vi "LINX - BlinkM Smart LED.vi"() -> ()   [LabVIEW 2020]
doc: "Set the color of a BlinkM Smart LED."
uses:
  vi.lib/MakerHub/LINX/LMH-LINX.lvlib
  vi.lib/MakerHub/LINX/Private/Device/Device.lvlib
  vi.lib/MakerHub/LINX/Public/Sensors/Lights/BlinkM/BlinkM.lvlib
  vi.lib/MakerHub/LINX/Public/Utilities/Open Serial.vi
panel:
  in  "I2C Channel":u8
  out "Loop Rate (Hz)":u32
  in  "Serial Port":refnum<visa-resource-name>
  in  "Stop Button":bool
  out "LED Color":u32(colorbox)
  in  "Blue":u8(slide) scale=0.0..255.0
  in  "Green":u8(slide) scale=0.0..255.0
  in  "Red":u8(slide) scale=0.0..255.0
  # "Circuit Schematic"
  # "LINX Device Settings"
  # "BlinkM Color"
  # "BlinkM Smart LED Example\n\nThis example demonstrates how to set the color of a BlinkM smart LED and assumes\nthe BlinkM is connected to I2C channel 0 and is the only device on the bus.\n\nNote: This example is configured to use a serial interface but can easily be modified\nto use TCP or run on myRIO.\n\nInstructions\n1. Select the COM Port associated with the LINX Device.\n2. Click the Run Arrow.\n3. Adjust the Red Green and Blue sliders to change the BlinkM color."
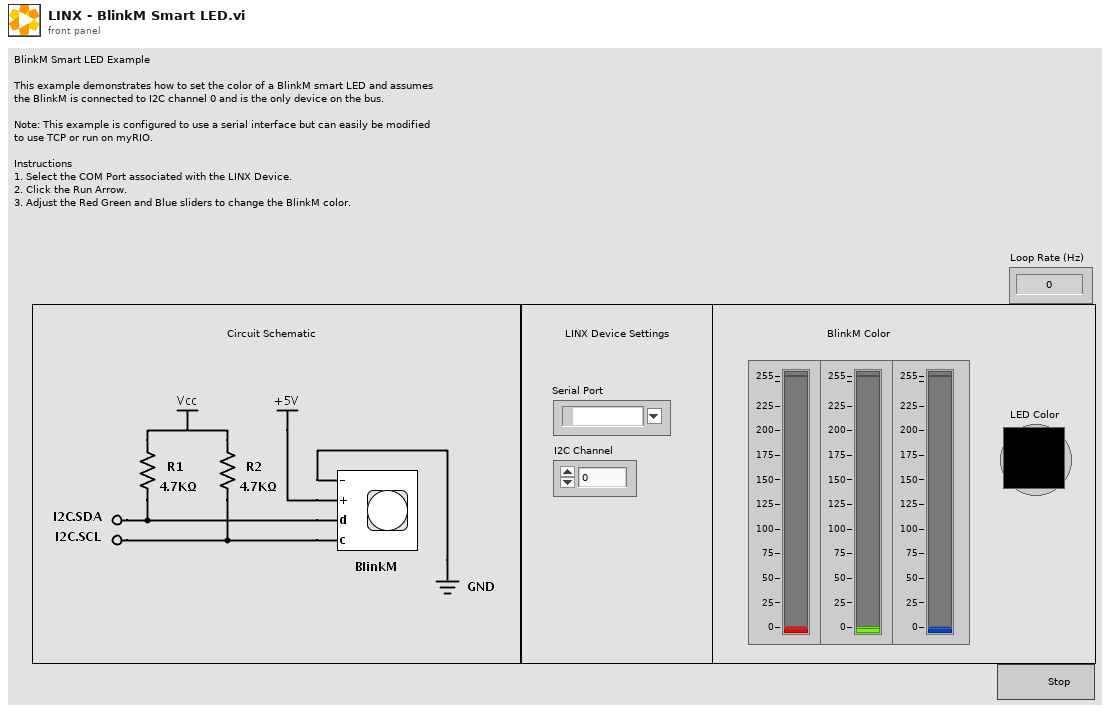
[diagram p1: front panel]
types:
  T1 = typedef "LMH-LINX.lvlib/LINX Ref.ctl" = cluster{"IO":T2, "Interface":T3, "LINX Device Config":T4}
  T2 = typedef "LMH-LINX.lvlib/Platform.ctl" = enum16{"Remote", "Local"}
  T3 = typedef "LMH-LINX.lvlib/Interface.ctl" = enum16{"Serial", "TCP"}
  T4 = typedef "Device.lvlib/LINX Device Config.ctl" = cluster{"Interface":T3, "COM Port":refnum<visa-resource-name>, "TCP Configuration":T5, "Device Family":u8, "Device ID":u8, "Device Name":string, "TCP Ref":refnum<k5>, "Channels":T6}
  T5 = typedef "Device.lvlib/TCP Config.ctl" = cluster{"IP Address":string, "Port":u16}
  T6 = typedef "LMH-LINX.lvlib/Channels.ctl" = cluster{"DI":u8[], "DO":u8[], "AI":u8[], "AO":u8[], "PWM":u8[], "QE":u8[], "UART":u8[], "I2C 2":u8[], "SPI":u8[], "CAN":u8[], "Servo":u8[], "AI Ref (V)":dbl, "AI Resolution (Bits)":u8, "AO Ref (V)":dbl, "AO Resolution (Bits)":u8}
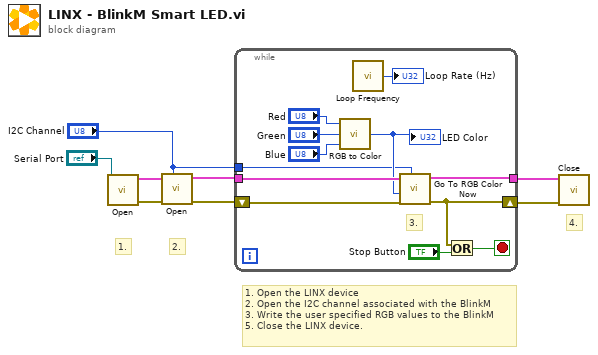
[diagram p0: block diagram]
diagram:
  # "4."
  # "2."
  # "1."
  # "1. Open the LINX device\n2. Open the I2C channel associated with the BlinkM\n3. Write the user specified RGB values to the BlinkM\n5. Close the LINX device."
  n1 = call-poly "Open.vi"("Serial Port"="Serial Port") -> ("Error Out"=w4:errorcluster, "LINX Resource"=w5:T1)  [unwired: 8 in, 1 out]
  n2 = call "Open.vi"("I2C Channel (0)"="I2C Channel", "Error In"=w4, "LINX Resource"=w5) -> ("Error Out"=w2:errorcluster, "LINX Resource"=w3:T1)  [unwired: 7 in]
  n3 = while {
    tunnel: w3 -> [w15]
    tunnel: [w14] -> w7
    shift-right: [w16] -> w8
    shift-left: w2 -> [w17]
    tunnel: "I2C Channel" -> [w9]
    stop <- w20 stop-if-true
    # "3."
    n4 = call <vilib>:"RGB to Color.vi"("B"="Blue", "G"="Green", "R"="Red") -> ("Color"=w13:u32)
    "LED Color" <- w13
    n5 = call "Loop Frequency.vi"() -> ("Loop Rate (Hz)"=→"Loop Rate (Hz)":u32)
    n6 = call "Go To RGB Color Now.vi"("I2C Channel (0)"=w9, "Error In"=w17, "Color"=w13, "LINX Resource"=w15) -> ("Error Out"=w16:errorcluster, "LINX Resource"=w14:T1)  [unwired: 6 in]
    n7 = Or(x=w16, y="Stop Button") -> (x .or. y?=w20:bool)
  }
  n8 = call "Close.vi"("Error In"=w8, "LINX Resource"=w7) -> ()  [unwired: 9 in, 1 out]
